vi "Base Test VI.vi"(10 "String Input":string, 11 "Numeric Input":i32) -> (1 "String Length":i32, 2 "String Output":string, 3 "Numeric Output":i32)   [LabVIEW 2020]
doc: "Base Test VI with elements for testing. Breakpoints and Probes must be set during tests using VI Scripting."
panel:
  out "Boolean Output":bool
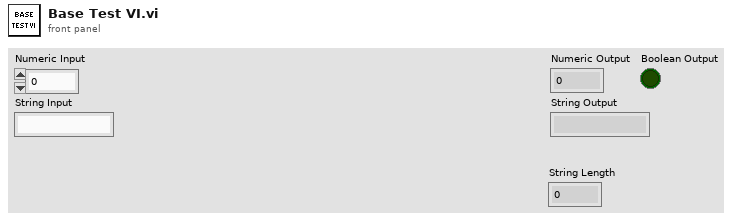
[diagram p1: front panel]
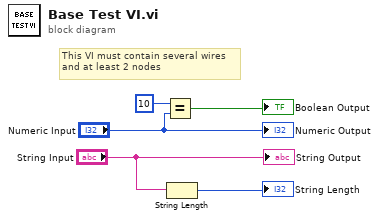
[diagram p0: block diagram]
diagram:
  # "This VI must contain several wires\nand at least 2 nodes"
  n1 = Equal?(x=10, y="Numeric Input") -> (x = y?=→"Boolean Output":bool)
  n2 = String Length(string="String Input") -> (length=→"String Length":i32)
  "Numeric Output" <- "Numeric Input"
  "String Output" <- "String Input"
